vi "runTestScenario.vi"(8 "error in (no error)":errorcluster, 11 "Device Configuration Test  in":refnum<class "Device Configuration Test.lvclass">) -> (0 "error out":errorcluster, 2 "TestExecution":T1, 3 "Device Configuration Test out":refnum<class "Device Configuration Test.lvclass">)   [LabVIEW 2015, in "Device Configuration Test.lvclass"]
uses:
  Device Configuration Test.lvclass
  Typedefs/TestExecution.ctl
  Device Configuration Test.lvclass/Device Configuration Test.ctl
  Typedefs/WriteLogMessageInput.ctl
  Typedefs/TestScenarioTypes.ctl
  Typedefs/PassFailTest.ctl
  Model/TestLog/ITestLog/ITestLog.lvclass
  Typedefs/ILCBTTypedefs.lvlib
  <userlib>/Common/ilc/ILC/ILC.lvclass
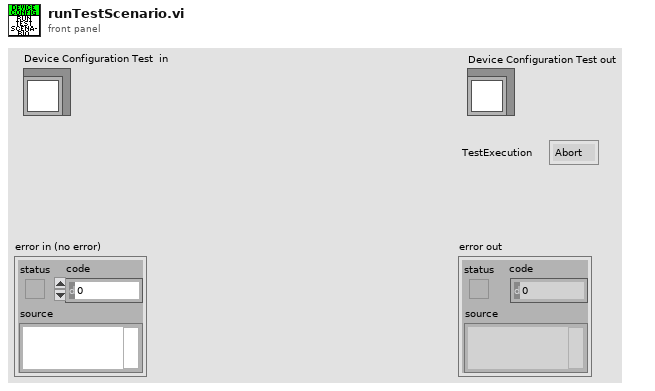
[diagram p1: front panel]
types:
  T1 = typedef "ILCBTTypedefs.lvlib/TestExecution.ctl" = enum16{"Abort", "Continue"}
  T2 = typedef "ILCBTTypedefs.lvlib/WriteLogMessageInput.ctl" = cluster{"Test Scenario":T3, "Description":string, "Actual Value":string, "Data File":string, "Result":T4}
  T3 = typedef "ILCBTTypedefs.lvlib/TestScenarioTypes.ctl" = enum16{"+3.3VA Supply Test", "+3.3VD Supply Test", "+5VA Supply Test", "+5VD Supply Test", "Unique ID Test", "TEDS Status Test", "LIMSW1_TTL Low Test", "LIMSW1_TTL High Test", "LIMSW2_TTL Low Test", "LIMSW2_TTL High Test", "Tachometer Test", "SSR_TTL Low Test", "SSR_TTL High Test", "SM_GPI Low Test", "SM_GPI High Test", "CW Motion Without Limit Test", "CW Motion With Limit Test", "CW Motion With Both Limits Test", "CW Motion on CCW Limit Test", "CCW Motion Without Limit Test", "CCW Motion With Limit Test", "CCW Motion With Both Limits Test", "CCW Motion on CW Limit Test", "RS232-TXD Low Test", "RS232-TXD High Test", "RS232-RTS Low Test", "RS232-RTS High Test", "RS232-RXD Low Test", "RS232-RXD High Test", "RS232-CTS Low Test", "RS232-CTS High Test", "Out_SS Low Test", "Out_SS High Test", "Out_SDI Low Test", "Out_SDI High Test", "Out_SCLK Low Test", "Out_SCLK High Test", "Reset Low Test", "Reset High Test", "1 Channel ADC Test", "3 Channel ADC Test", "5 Channel ADC Test", "Vref Test", "ROT Test", "DAC1 Test", "DAC2 Test", "DAC3 Test", "DAC4 Test", "BIAS Test", "EXC1 Test", "EXC2 Test", "EXC3 Test", "EXC4 Test"}
  T4 = typedef "ILCBTTypedefs.lvlib/PassFailTest.ctl" = enum16{"Fail", "Pass", "NA"}
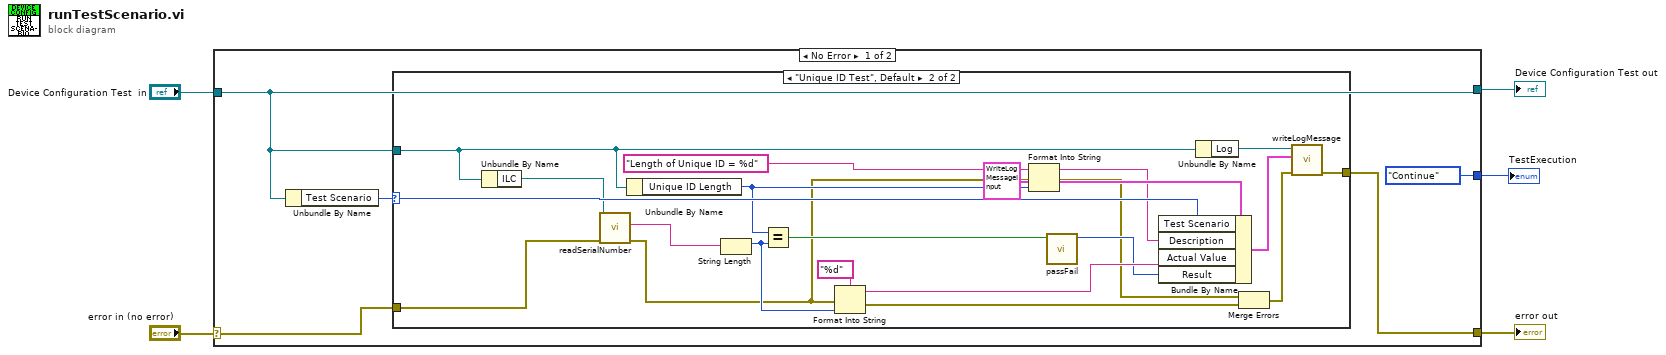
[diagram p0: block diagram]
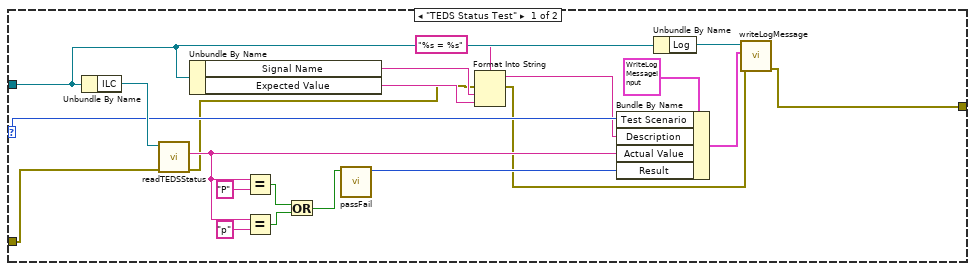
[diagram p2: hidden frame]
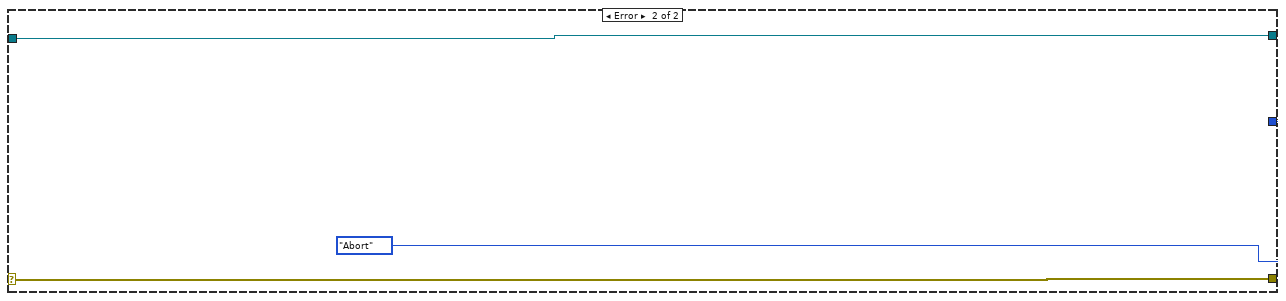
[diagram p3: hidden frame]
diagram:
  n1 = case shown="No Error" "error in (no error)" {
    selector: "error in (no error)" -> [w8 w55]
    tunnel: [w6 w55] -> w4
    tunnel: [TestExecution."Continue" ("TestExecution") TestExecution."Abort" ("TestExecution")] -> w3
    tunnel: "Device Configuration Test  in" -> [w7 w53]
    tunnel: [w7 w53] -> w1
    frame No Error {
      n2 = Unbundle By Name(w7) -> ("Test Scenario"=w9:T3)
      n3 = case shown="\"Unique ID Test\", Default" w9 {
        selector: w9 -> [w19 w45]
        tunnel: w7 -> [w17 w39]
        tunnel: w8 -> [w27 w52]
        tunnel: [w18 w40] -> w6
        frame "TEDS Status Test" {
          n4 = Unbundle By Name(w17) -> ("ILC"=w28:refnum<class "ILC.lvclass">)
          n5 = call <userlib>:"readTEDSStatus.vi"("error in (no error)"=w27, "ILC in"=w28) -> ("error out"=w12:errorcluster, "TEDS Status"=w21:string)  [unwired: 7 in, 1 out]
          n6 = Unbundle By Name(w17) -> ("Signal Name"=w15:string, "Expected Value"=w14:string)
          n7 = Equal?(x=w21, y="P") -> (x = y?=w24:bool)
          n8 = Equal?(x=w21, y="p") -> (x = y?=w20:bool)
          n9 = Or(x=w24, y=w20) -> (x .or. y?=w23:bool)
          n10 = call "passFail.vi"("Boolean"=w23) -> ("Result"=w30:T4)  [unwired: 10 in]
          n11 = Format Into String(format string="%s = %s", error in=w12, w15, w14) -> (resulting string=w13:string, error out=w11:errorcluster)  [unwired: 1 in]
          n12 = Bundle By Name(cluster=T2 {"Test Scenario"=enum."+3.3VA Supply Test", "Description"="", "Actual Value"="", "Data File"="", "Result"=enum."Fail"} ("WriteLogMessageInput"), "Test Scenario"=w19, "Description"=w13, "Actual Value"=w21, "Result"=w30) -> (w29:T2)
          n13 = Unbundle By Name(w17) -> ("Log"=w26:refnum<class "ITestLog.lvclass">)
          n14 = call-dynamic "writeLogMessage.vi"("error in (no error)"=w11, "WriteLogMessageInput"=w29, "ITestLog in"=w26) -> ("error out"=w18:errorcluster)  [unwired: 7 in, 1 out]
        }
        frame "Unique ID Test", Default {
          n15 = Unbundle By Name(w39) -> ("ILC"=w42:refnum<class "ILC.lvclass">)
          n16 = call <userlib>:"readSerialNumber.vi"("error in (no error)"=w52, "ILC in"=w42) -> ("error out"=w35:errorcluster, "Serial Number"=w48:string)  [unwired: 7 in, 1 out]
          n17 = Unbundle By Name(w39) -> ("Unique ID Length"=w36:u8)
          n18 = String Length(string=w48) -> (length=w47:i32)
          n19 = Equal?(x=w36, y=w47) -> (x = y?=w44:bool)
          n20 = Format Into String(format string="%d", error in=w35, w47) -> (resulting string=w46:string, error out=w33:errorcluster)  [unwired: 1 in]
          n21 = Format Into String(format string="Length of Unique ID = %d" ("Description"), error in=w35, w36) -> (resulting string=w38:string, error out=w32:errorcluster)  [unwired: 1 in]
          n22 = call "passFail.vi"("Boolean"=w44) -> ("Result"=w43:T4)  [unwired: 10 in]
          n23 = Bundle By Name(cluster=T2 {"Test Scenario"=enum."+3.3VA Supply Test", "Description"="", "Actual Value"="", "Data File"="", "Result"=enum."Fail"} ("WriteLogMessageInput"), "Test Scenario"=w45, "Description"=w38, "Actual Value"=w46, "Result"=w43) -> (w41:T2)
          n24 = Unbundle By Name(w39) -> ("Log"=w51:refnum<class "ITestLog.lvclass">)
          n25 = Merge Errors(w32, w33) -> (w34:errorcluster)
          n26 = call-dynamic "writeLogMessage.vi"("error in (no error)"=w34, "WriteLogMessageInput"=w41, "ITestLog in"=w51) -> ("error out"=w40:errorcluster)  [unwired: 7 in, 1 out]
        }
      }
    }
    frame Error {
    }
  }
  "Device Configuration Test out" <- w1
  "error out" <- w4
  "TestExecution" <- w3
